vi "Build Report String.vi"(8 "error in (no error)":errorcluster, 10 "Report Data":T1, 11 "Boolean Assertion in":refnum<class "Boolean Assertion.lvclass">) -> (0 "error out":errorcluster, 2 "Report String":string, 3 "Boolean Assertion out":refnum<class "Boolean Assertion.lvclass">)   [LabVIEW 2020, in "MacroAssert.lvlib" / "Boolean Assertion.lvclass"]
doc: "Builds a string using <B>Step</B> and <B>Report Data</B> to be included in a report."
uses:
  Boolean Assertion.lvclass
  CTLs/Report Data.ctl
  Assertion Step/Assertion Step.lvclass
  MacroAssert.lvlib
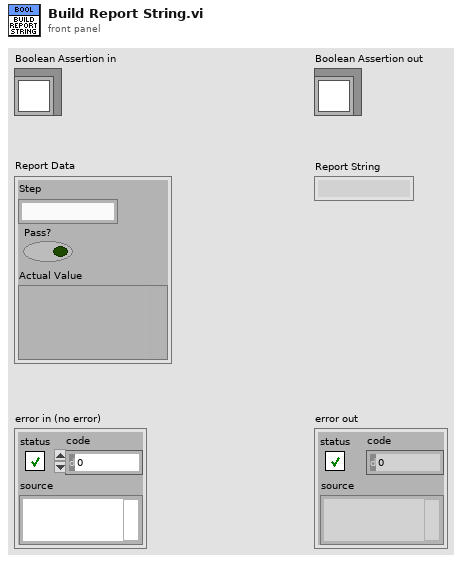
[diagram p1: front panel]
types:
  T1 = typedef "MacroAssert.lvlib/Report Data.ctl" = cluster{"Step":string, "Pass?":bool, "Actual Value":variant}
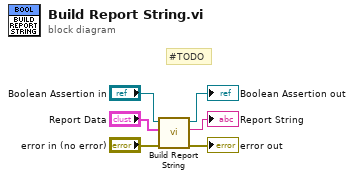
[diagram p0: block diagram]
diagram:
  # "#TODO"
  n1 = call-parent "Build Report String.vi"("error in (no error)"="error in (no error)", "Report Data"="Report Data", "Step in"="Boolean Assertion in") -> ("error out"=→"error out":errorcluster, "Report String"=→"Report String":string, "Step out"=→"Boolean Assertion out":refnum<class "Boolean Assertion.lvclass">)  [unwired: 6 in]
